vi "Swerve Begin.vi"   [LabVIEW 2016]
uses:
  <vilib>/Rock Robotics/WPI/Counter/WPI_CounterDigitalInputToDigitalSource.vi
  <vilib>/Rock Robotics/SystemInterfaces/DIO/FPGA_DIOChannel.ctl
  <vilib>/Rock Robotics/WPI/Switch/WPI_SwitchOpenLimit.vi
  <vilib>/Rock Robotics/WPI/MotorControl/WPI_MotorControlOpen Talon.vi
  <vilib>/Rock Robotics/WPI/CAN/TalonSRX/WPI_CANTalonSRX_APIControlMode.ctl
  <vilib>/Rock Robotics/WPI/CAN/TalonSRX/WPI_CANTalonSRX_BrakeOverride.ctl
types:
  T1 = typedef "WPI_CANTalonSRX_BrakeOverride.ctl" = enum8{"No Override", "Override to Coast", "Override to Brake"}
  T2 = typedef "FPGA_DIOChannel.ctl" = enum8{"DIO 0", "DIO 1", "DIO 2", "DIO 3", "DIO 4", "DIO 5", "DIO 6", "DIO 7", "DIO 8", "DIO 9", "DIO MXP 0", "DIO MXP 1", "DIO MXP 2", "DIO MXP 3", "DIO MXP 4", "DIO MXP 5", "DIO MXP 6", "DIO MXP 7", "DIO MXP 8", "DIO MXP 9", "DIO MXP 10", "DIO MXP 11", "DIO MXP 12", "DIO MXP 13", "DIO MXP 14", "DIO MXP 15", "SPI Port CS1", "SPI Port CS2", "SPI Port CS3", "SPI Port MISO", "SPI Port MOSI", "Invalid"}
  T3 = typedef "WPI_CANTalonSRX_APIControlMode.ctl" = enum8{"Percent VBus", "Speed", "Position", "Slave", "Unchanged / Invalid", "Voltage Compensation", "Current", "Motion Profile"}
  T4 = typedef "WPI_SwitchDevRef.ctl" = cluster{"DevStatus":errorcluster, "DIO Channel":T2, "CntIndex":T5, "Normally Closed":bool}
  T5 = typedef "FPGA_CounterCtrSystemIndex.ctl" = enum8{"Ctr 0", "Ctr 1", "Ctr 2", "Ctr 3", "Ctr 4", "Ctr 5", "Ctr 6", "Ctr 7", "Invalid"}
  T6 = typedef "WPI_DigitalInputDevRef.ctl" = cluster{"DevStatus":errorcluster, "DIO Channel":T2}
  T7 = typedef "FPGA_CounterEncoderSourceConvertionLVSourceType.ctl" = cluster{"DevStatus":errorcluster, "AnalogTriggerMode?":bool, "DigitalMode":cluster{"DIO Channel":T8}, "AnalogTriggerMode":cluster{"AnalogTriggerIndex":T9, "OutputType":T10}}
  T8 = typedef "FPGA_DIODigitalSourceChannel.ctl" = enum8{"DIO 0", "DIO 1", "DIO 2", "DIO 3", "DIO 4", "DIO 5", "DIO 6", "DIO 7", "DIO 8", "DIO 9", "DIO MXP 0", "DIO MXP 1", "DIO MXP 2", "DIO MXP 3", "DIO MXP 4", "DIO MXP 5", "DIO MXP 6", "DIO MXP 7", "DIO MXP 8", "DIO MXP 9", "DIO MXP 10", "DIO MXP 11", "DIO MXP 12", "DIO MXP 13", "DIO MXP 14", "DIO MXP 15", "Disabled"}
  T9 = typedef "FPGA_AnalogTriggerIndex.ctl" = enum8{"Trig 0", "Trig 1", "Trig 2", "Trig 3", "Trig 4", "Trig 5", "Trig 6", "Trig 7", "Invalid"}
  T10 = typedef "FPGA_AnalogTriggerOutType.ctl" = enum16{"InWindow", "TriggerState", "Rising", "Falling"}
  T11 = typedef "WPI_MotorControlDeviceRef.ctl" = cluster{"DeviceStatus":errorcluster, "Type":T12, "PWM":cluster{"PWM Channel":T13, "DeadBand":T14}, "CAN":cluster{"Device Number":u8, "SetOutput VI Ref":variant, "GetOutput VI Ref":variant, "Enable VI Ref":variant, "Disable VI Ref":variant, "Data":variant}, "Invert":bool}
  T12 = typedef "WPI_MotorControlType.ctl" = enum16{"PWM", "CAN"}
  T13 = typedef "FPGA_DIOPWMChannel.ctl" = enum8{"PWM 0", "PWM 1", "PWM 2", "PWM 3", "PWM 4", "PWM 5", "PWM 6", "PWM 7", "PWM 8", "PWM 9", "PWM MXP 0", "PWM MXP 1", "PWM MXP 2", "PWM MXP 3", "PWM MXP 4", "PWM MXP 5", "PWM MXP 6", "PWM MXP 7", "PWM MXP 8", "PWM MXP 9", "Invalid"}
  T14 = typedef "WPI_PWMDeadband.ctl" = cluster{"Name":string, "maxPositivePwm":i32, "minPositivePwm":i32, "centerPwm":i32, "maxNegativePwm":i32, "minNegativePwm":i32, "angularRange":u16}
  T15 = typedef "WPI_EncoderDevRef.ctl" = cluster{"DevStatus":errorcluster, "EncoderIndex":T16, "CounterIndex":T5, "DistancePerCount":dbl, "Decoding Type":T17}
  T16 = typedef "FPGA_EncoderIdx.ctl" = enum8{"Enc 0", "Enc 1", "Enc 2", "Enc 3", "Enc 4", "Enc 5", "Enc 6", "Enc 7", "Invalid"}
  T17 = typedef "WPI_EncoderType.ctl" = enum16{"1x", "2x", "4x"}
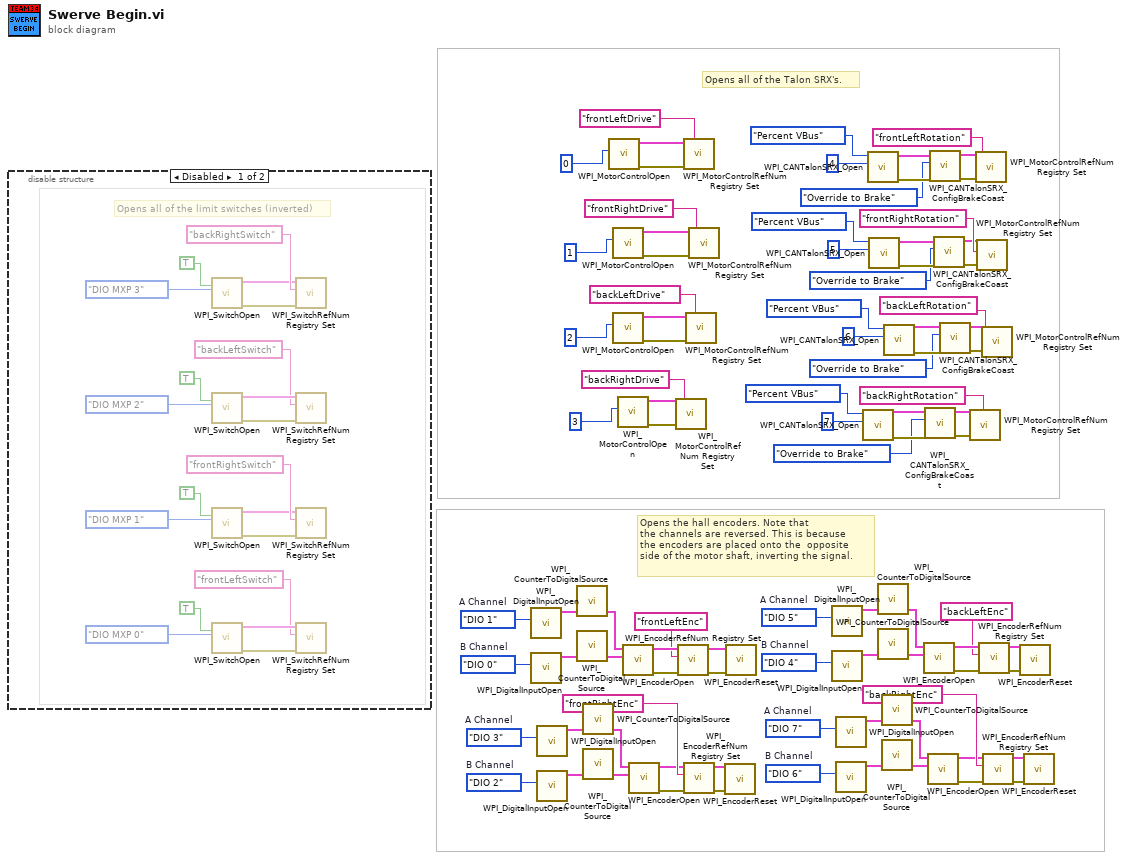
[diagram p0: block diagram]
diagram:
  w40 = FPGA_DIOChannel."DIO 6"  # B Channel
  w41 = FPGA_DIOChannel."DIO 7"  # A Channel
  w57 = FPGA_DIOChannel."DIO 4"  # B Channel
  w56 = FPGA_DIOChannel."DIO 5"  # A Channel
  w58 = FPGA_DIOChannel."DIO 2"  # B Channel
  w59 = FPGA_DIOChannel."DIO 3"  # A Channel
  w75 = FPGA_DIOChannel."DIO 0"  # B Channel
  w74 = FPGA_DIOChannel."DIO 1"  # A Channel
  # "Opens all of the Talon SRX's."
  # "Opens the hall encoders. Note that \nthe channels are reversed. This is because\nthe encoders are placed onto the  opposite\nside of the motor shaft, inverting the signal."
  n1 = disable-structure shown="Disabled" {
    frame Disabled {
      # "Opens all of the limit switches (inverted)"
      n2 = call-poly <vilib>:"WPI_SwitchOpen.vi"("Normally Closed"=TRUE, "DIO Channel"=FPGA_DIOChannel."DIO MXP 3") -> ("error out"=w97:errorcluster, "SwitchDevRef"=w98:T4)  [unwired: 8 in]
      n3 = call-poly <vilib>:"WPI_SwitchOpen.vi"("Normally Closed"=TRUE, "DIO Channel"=FPGA_DIOChannel."DIO MXP 2") -> ("error out"=w104:errorcluster, "SwitchDevRef"=w103:T4)  [unwired: 8 in]
      n4 = call-poly <vilib>:"WPI_SwitchOpen.vi"("Normally Closed"=TRUE, "DIO Channel"=FPGA_DIOChannel."DIO MXP 1") -> ("error out"=w105:errorcluster, "SwitchDevRef"=w106:T4)  [unwired: 8 in]
      n5 = call-poly <vilib>:"WPI_SwitchOpen.vi"("Normally Closed"=TRUE, "DIO Channel"=FPGA_DIOChannel."DIO MXP 0") -> ("error out"=w112:errorcluster, "SwitchDevRef"=w111:T4)  [unwired: 8 in]
      n6 = call <vilib>:"WPI_SwitchRefNum Registry Set.vi"("error in (no error)"=w97, "refnum name"="backRightSwitch", "SwitchDevRef"=w98) -> ()  [unwired: 7 in, 2 out]
      n7 = call <vilib>:"WPI_SwitchRefNum Registry Set.vi"("error in (no error)"=w104, "refnum name"="backLeftSwitch", "SwitchDevRef"=w103) -> ()  [unwired: 7 in, 2 out]
      n8 = call <vilib>:"WPI_SwitchRefNum Registry Set.vi"("error in (no error)"=w105, "refnum name"="frontRightSwitch", "SwitchDevRef"=w106) -> ()  [unwired: 7 in, 2 out]
      n9 = call <vilib>:"WPI_SwitchRefNum Registry Set.vi"("error in (no error)"=w112, "refnum name"="frontLeftSwitch", "SwitchDevRef"=w111) -> ()  [unwired: 7 in, 2 out]
    }
    frame Enabled {
    }
  }
  n10 = call <vilib>:"WPI_DigitalInputOpen.vi"("DIO Channel"=w74) -> ("DigitalInputDevRef"=w71:T6)  [unwired: 1 in, 9 out]
  n11 = call <vilib>:"WPI_DigitalInputOpen.vi"("DIO Channel"=w75) -> ("DigitalInputDevRef"=w72:T6)  [unwired: 1 in, 9 out]
  n12 = call <vilib>:"WPI_DigitalInputOpen.vi"("DIO Channel"=w59) -> ("DigitalInputDevRef"=w62:T6)  [unwired: 1 in, 9 out]
  n13 = call <vilib>:"WPI_DigitalInputOpen.vi"("DIO Channel"=w58) -> ("DigitalInputDevRef"=w61:T6)  [unwired: 1 in, 9 out]
  n14 = call-poly <vilib>:"WPI_CounterToDigitalSource.vi"("DigitalInputDevRef"=w71) -> ("Digital Source"=w70:T7)  [unwired: 6 out]
  n15 = call-poly <vilib>:"WPI_CounterToDigitalSource.vi"("DigitalInputDevRef"=w72) -> ("Digital Source"=w73:T7)  [unwired: 6 out]
  n16 = call-poly <vilib>:"WPI_CounterToDigitalSource.vi"("DigitalInputDevRef"=w62) -> ("Digital Source"=w63:T7)  [unwired: 6 out]
  n17 = call-poly <vilib>:"WPI_CounterToDigitalSource.vi"("DigitalInputDevRef"=w61) -> ("Digital Source"=w60:T7)  [unwired: 6 out]
  n18 = call-poly <vilib>:"WPI_MotorControlOpen.vi"("PWM Channel"=u8 0 ("Device Number")) -> ("error out"=w1:errorcluster, "MotorControlDeviceRef"=w2:T11)  [unwired: 9 in]
  n19 = call-poly <vilib>:"WPI_MotorControlOpen.vi"("PWM Channel"=u8 1 ("Device Number")) -> ("error out"=w3:errorcluster, "MotorControlDeviceRef"=w4:T11)  [unwired: 9 in]
  n20 = call-poly <vilib>:"WPI_MotorControlOpen.vi"("PWM Channel"=u8 2 ("Device Number")) -> ("error out"=w5:errorcluster, "MotorControlDeviceRef"=w6:T11)  [unwired: 9 in]
  n21 = call-poly <vilib>:"WPI_MotorControlOpen.vi"("PWM Channel"=u8 3 ("Device Number")) -> ("error out"=w30:errorcluster, "MotorControlDeviceRef"=w31:T11)  [unwired: 9 in]
  n22 = call <vilib>:"WPI_EncoderOpen.vi"("BSource"=w73, "ASource"=w70) -> ("error out"=w69:errorcluster, "EncoderDevRef"=w68:T15)  [unwired: 6 in, 2 out]
  n23 = call <vilib>:"WPI_EncoderOpen.vi"("BSource"=w60, "ASource"=w63) -> ("error out"=w64:errorcluster, "EncoderDevRef"=w65:T15)  [unwired: 6 in, 2 out]
  n24 = call <vilib>:"WPI_MotorControlRefNum Registry Set.vi"("error in (no error)"=w30, "refnum name"="backRightDrive", "MotorControlDevRef"=w31) -> ()  [unwired: 7 in, 2 out]
  n25 = call <vilib>:"WPI_EncoderRefNum Registry Set.vi"("error in (no error)"=w69, "refnum name"="frontLeftEnc", "EncoderDevRef"=w68) -> ("error out"=w39:errorcluster, "EncoderDevRef"=w38:T15)  [unwired: 7 in]
  n26 = call <vilib>:"WPI_MotorControlRefNum Registry Set.vi"("error in (no error)"=w1, "refnum name"="frontLeftDrive", "MotorControlDevRef"=w2) -> ()  [unwired: 7 in, 2 out]
  n27 = call <vilib>:"WPI_EncoderRefNum Registry Set.vi"("error in (no error)"=w64, "refnum name"="frontRightEnc", "EncoderDevRef"=w65) -> ("error out"=w36:errorcluster, "EncoderDevRef"=w37:T15)  [unwired: 7 in]
  n28 = call <vilib>:"WPI_MotorControlRefNum Registry Set.vi"("error in (no error)"=w5, "refnum name"="backLeftDrive", "MotorControlDevRef"=w6) -> ()  [unwired: 7 in, 2 out]
  n29 = call <vilib>:"WPI_MotorControlRefNum Registry Set.vi"("error in (no error)"=w3, "refnum name"="frontRightDrive", "MotorControlDevRef"=w4) -> ()  [unwired: 7 in, 2 out]
  n30 = call <vilib>:"WPI_EncoderReset.vi"("error in (no error)"=w36, "EncoderDevRef"=w37) -> ()  [unwired: 8 in, 2 out]
  n31 = call <vilib>:"WPI_EncoderReset.vi"("error in (no error)"=w39, "EncoderDevRef"=w38) -> ()  [unwired: 8 in, 2 out]
  n32 = call <vilib>:"WPI_DigitalInputOpen.vi"("DIO Channel"=w56) -> ("DigitalInputDevRef"=w53:T6)  [unwired: 1 in, 9 out]
  n33 = call <vilib>:"WPI_DigitalInputOpen.vi"("DIO Channel"=w57) -> ("DigitalInputDevRef"=w54:T6)  [unwired: 1 in, 9 out]
  n34 = call <vilib>:"WPI_DigitalInputOpen.vi"("DIO Channel"=w41) -> ("DigitalInputDevRef"=w44:T6)  [unwired: 1 in, 9 out]
  n35 = call <vilib>:"WPI_DigitalInputOpen.vi"("DIO Channel"=w40) -> ("DigitalInputDevRef"=w43:T6)  [unwired: 1 in, 9 out]
  n36 = call <vilib>:"WPI_CANTalonSRX_Open.vi"("Device Number"=u8 7, "Control Mode"=WPI_CANTalonSRX_APIControlMode."Percent VBus") -> ("error out"=w9:errorcluster, "CAN Talon SRX Ref"=w10:T11)  [unwired: 8 in]
  n37 = call <vilib>:"WPI_CANTalonSRX_Open.vi"("Device Number"=u8 4, "Control Mode"=WPI_CANTalonSRX_APIControlMode."Percent VBus") -> ("error out"=w24:errorcluster, "CAN Talon SRX Ref"=w25:T11)  [unwired: 8 in]
  n38 = call <vilib>:"WPI_CANTalonSRX_Open.vi"("Device Number"=u8 5, "Control Mode"=WPI_CANTalonSRX_APIControlMode."Percent VBus") -> ("error out"=w19:errorcluster, "CAN Talon SRX Ref"=w20:T11)  [unwired: 8 in]
  n39 = call-poly <vilib>:"WPI_CounterToDigitalSource.vi"("DigitalInputDevRef"=w53) -> ("Digital Source"=w52:T7)  [unwired: 6 out]
  n40 = call-poly <vilib>:"WPI_CounterToDigitalSource.vi"("DigitalInputDevRef"=w54) -> ("Digital Source"=w55:T7)  [unwired: 6 out]
  n41 = call-poly <vilib>:"WPI_CounterToDigitalSource.vi"("DigitalInputDevRef"=w44) -> ("Digital Source"=w45:T7)  [unwired: 6 out]
  n42 = call-poly <vilib>:"WPI_CounterToDigitalSource.vi"("DigitalInputDevRef"=w43) -> ("Digital Source"=w42:T7)  [unwired: 6 out]
  n43 = call <vilib>:"WPI_CANTalonSRX_Open.vi"("Device Number"=u8 6, "Control Mode"=WPI_CANTalonSRX_APIControlMode."Percent VBus") -> ("error out"=w14:errorcluster, "CAN Talon SRX Ref"=w15:T11)  [unwired: 8 in]
  n44 = call <vilib>:"WPI_EncoderOpen.vi"("BSource"=w55, "ASource"=w52) -> ("error out"=w51:errorcluster, "EncoderDevRef"=w50:T15)  [unwired: 6 in, 2 out]
  n45 = call <vilib>:"WPI_CANTalonSRX_ConfigBrakeCoast.vi"("error in (no error)"=w9, "Brake / Coast Mode"=WPI_CANTalonSRX_BrakeOverride."Override to Brake", "CAN Talon SRX Ref"=w10) -> ("error out"=w12:errorcluster, "CAN Talon SRX Ref"=w11:T11)  [unwired: 7 in]
  n46 = call <vilib>:"WPI_EncoderOpen.vi"("BSource"=w42, "ASource"=w45) -> ("error out"=w46:errorcluster, "EncoderDevRef"=w47:T15)  [unwired: 6 in, 2 out]
  n47 = call <vilib>:"WPI_CANTalonSRX_ConfigBrakeCoast.vi"("error in (no error)"=w24, "Brake / Coast Mode"=WPI_CANTalonSRX_BrakeOverride."Override to Brake", "CAN Talon SRX Ref"=w25) -> ("error out"=w27:errorcluster, "CAN Talon SRX Ref"=w26:T11)  [unwired: 7 in]
  n48 = call <vilib>:"WPI_CANTalonSRX_ConfigBrakeCoast.vi"("error in (no error)"=w19, "Brake / Coast Mode"=WPI_CANTalonSRX_BrakeOverride."Override to Brake", "CAN Talon SRX Ref"=w20) -> ("error out"=w22:errorcluster, "CAN Talon SRX Ref"=w21:T11)  [unwired: 7 in]
  n49 = call <vilib>:"WPI_CANTalonSRX_ConfigBrakeCoast.vi"("error in (no error)"=w14, "Brake / Coast Mode"=WPI_CANTalonSRX_BrakeOverride."Override to Brake", "CAN Talon SRX Ref"=w15) -> ("error out"=w17:errorcluster, "CAN Talon SRX Ref"=w16:T11)  [unwired: 7 in]
  n50 = call <vilib>:"WPI_MotorControlRefNum Registry Set.vi"("error in (no error)"=w12, "refnum name"="backRightRotation", "MotorControlDevRef"=w11) -> ()  [unwired: 7 in, 2 out]
  n51 = call <vilib>:"WPI_MotorControlRefNum Registry Set.vi"("error in (no error)"=w27, "refnum name"="frontLeftRotation", "MotorControlDevRef"=w26) -> ()  [unwired: 7 in, 2 out]
  n52 = call <vilib>:"WPI_MotorControlRefNum Registry Set.vi"("error in (no error)"=w22, "refnum name"="frontRightRotation", "MotorControlDevRef"=w21) -> ()  [unwired: 7 in, 2 out]
  n53 = call <vilib>:"WPI_EncoderRefNum Registry Set.vi"("error in (no error)"=w51, "refnum name"="backLeftEnc", "EncoderDevRef"=w50) -> ("error out"=w33:errorcluster, "EncoderDevRef"=w32:T15)  [unwired: 7 in]
  n54 = call <vilib>:"WPI_MotorControlRefNum Registry Set.vi"("error in (no error)"=w17, "refnum name"="backLeftRotation", "MotorControlDevRef"=w16) -> ()  [unwired: 7 in, 2 out]
  n55 = call <vilib>:"WPI_EncoderRefNum Registry Set.vi"("error in (no error)"=w46, "refnum name"="backRightEnc", "EncoderDevRef"=w47) -> ("error out"=w35:errorcluster, "EncoderDevRef"=w34:T15)  [unwired: 7 in]
  n56 = call <vilib>:"WPI_EncoderReset.vi"("error in (no error)"=w33, "EncoderDevRef"=w32) -> ()  [unwired: 8 in, 2 out]
  n57 = call <vilib>:"WPI_EncoderReset.vi"("error in (no error)"=w35, "EncoderDevRef"=w34) -> ()  [unwired: 8 in, 2 out]
